vi "Auto Config Core.vi"(5 "Protected Signal GUID":string="D95BE1B9-793B-430A-998F-7F352C03EC7C", 6 "Protection Value GUID":string, 7 "Counter Value GUID":string="94e87467-031b-484c-a85e-bcbac581524d", 8 "error in (no error)":errorcluster, 9 "Signal Page GUID":string, 10 "Auto Config Setting":T1={"Rolling Counter"=FALSE, "RC Matching Strings"=[], "CRC"=FALSE, "CRC Matching Strings"=[], "Rolling Counter Max Count"=15.0, "Protection Type Number"=4}, 11 "Node Ptr":T2 format="%.0x") -> (0 "error out":errorcluster)   [LabVIEW 2023, in "Protection and Counter Support System Explorer.lvlib"]
uses:
  Protection and Counter Support System Explorer.lvlib
  <vilib>/NI VeriStand/Custom Device API/Custom Device Item Ref.ctl
  Types/Auto Config Setting.ctl
  <vilib>/NI VeriStand/Custom Device Tools/Custom Device Utility Library/Custom Device Utility Library.lvlib
  <vilib>/NI VeriStand/Custom Device API/Custom Device API.lvlib
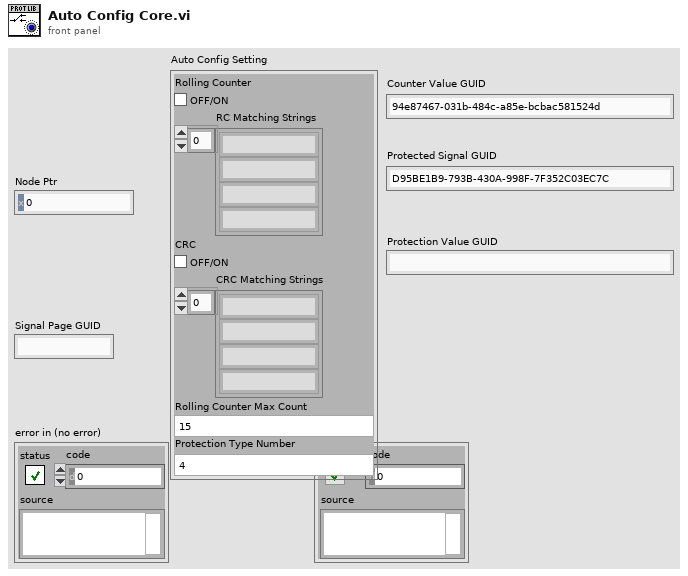
[diagram p1: front panel]
types:
  T1 = typedef "Protection and Counter Support System Explorer.lvlib/Auto Config Setting.ctl" = cluster{"Rolling Counter":bool, "RC Matching Strings":string[], "CRC":bool, "CRC Matching Strings":string[], "Rolling Counter Max Count":dbl, "Protection Type Number":u8}
  T2 = typedef "Custom Device API.lvlib/Custom Device Item Ref.ctl" = u64
  T3 = typedef "Custom Device API.lvlib/Custom Device Item Info.ctl" = cluster{"Name":string, "Is Channel":bool, "GUID":string, "Is Waveform":bool}
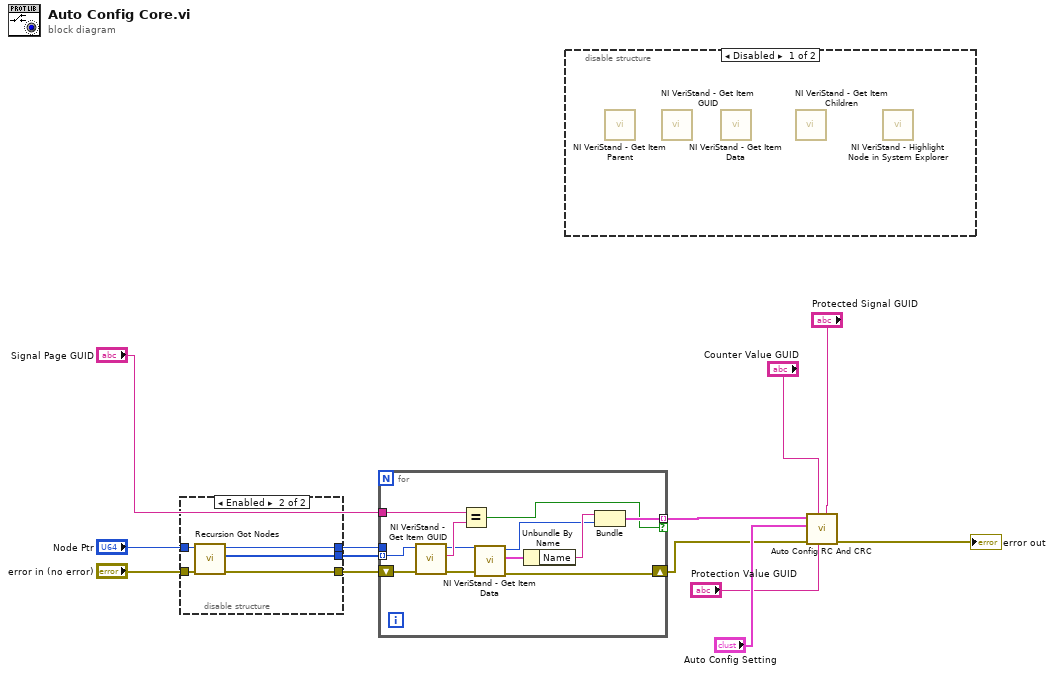
[diagram p0: block diagram]
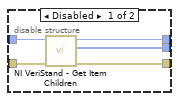
[diagram p2: hidden frame]
diagram:
  n1 = disable-structure shown="Enabled" {
    disable-tunnel: "Node Ptr" -> [w18 w23]
    disable-tunnel: "error in (no error)" -> [w17 w20]
    disable-tunnel: [w16 w19] -> w11
    disable-tunnel: [w15 w22] -> w10
    disable-tunnel: [w14 w21] -> w8
    frame Disabled {
      n2 = call <vilib>:"NI VeriStand - Get Item Children.vi"("error in (no error)"=w17, "Item Ref in"=w18) -> ("error out"=w16:errorcluster, "Child Refs"=w14:T2[], "Item Ref out"=w15:T2)  [unwired: 6 in, 1 out]
    }
    frame Enabled {
      n3 = call "Recursion Got Nodes.vi"("error in (no error)"=w20, "Node Ptr"=w23) -> ("error out"=w19:errorcluster, "Array"=w21:T2[], "Node Ptr"=w22:T2)  [unwired: 7 in]
    }
  }
  n4 = for {
    tunnel: w10 -> [_]
    tunnel: "Signal Page GUID" -> [w33]
    tunnel: w8 -> [w32] mode=indexing
    shift-right: [w30] -> w5
    shift-left: w11 -> [w35]
    tunnel: [w25] -> w7 mode=indexing if=w24
    n5 = call <vilib>:"NI VeriStand - Get Item GUID.vi"("error in (no error)"=w35, "Item Ref in"=w32) -> ("error out"=w31:errorcluster, "GUID"=w34:string, "Item Ref out"=w29:T2)  [unwired: 7 in]
    n6 = Equal?(x=w33, y=w34) -> (x = y?=w24:bool)
    n7 = call <vilib>:"NI VeriStand - Get Item Data.vi"("error in (no error)"=w31, "Item Ref in"=w29) -> ("error out"=w30:errorcluster, "Item Info"=w28:T3, "Item Ref out"=w26:T2)  [unwired: 6 in, 1 out]
    n8 = Unbundle By Name(w28) -> ("Name"=w27:string)
    n9 = Bundle("Name"=w27, "Item Ref out"=w26) -> (w25:cluster{"Name":string, "Item Ref out":T2})  [unwired: 1 in]
  }
  n10 = disable-structure shown="Disabled" {
    frame Disabled {
      n11 = call <vilib>:"NI VeriStand - Get Item Parent.vi"() -> ()  [unwired: 8 in, 4 out]
      n12 = call <vilib>:"NI VeriStand - Get Item GUID.vi"() -> ()  [unwired: 9 in, 3 out]
      n13 = call <vilib>:"NI VeriStand - Get Item Data.vi"() -> ()  [unwired: 8 in, 4 out]
      n14 = call <vilib>:"NI VeriStand - Get Item Children.vi"() -> ()  [unwired: 8 in, 4 out]
      n15 = call <vilib>:"NI VeriStand - Highlight Node in System Explorer.vi"() -> ()  [unwired: 10 in, 2 out]
    }
    frame Enabled {
    }
  }
  n16 = call "Auto Config RC And CRC.vi"("Protected Signal GUID"="Protected Signal GUID", "Protection Value GUID"="Protection Value GUID", "Counter Value GUID"="Counter Value GUID", "error in (no error)"=w5, "Auto Config Setting"="Auto Config Setting", "Array"=w7) -> ("error out"=→"error out":errorcluster)  [unwired: 5 in]
